vi "Ballard - 1553 Asynchronous RT Driver VI.vi"(10 "Parameters":variant, 11 "Process":refnum<class "Process.lvclass">) -> ()   [LabVIEW 2017, in "Ballard MIL-1553 Engine.lvlib"]
doc: "This VI is the Asynchronous VI for RT part."
uses:
  Ballard MIL-1553 Engine.lvlib
  <vilib>/NI/NIVS Inline Async API/_VS Inline Async API/Process/Process.lvclass
  Controls/RT Async Data.ctl
  Controls/RT Async_Map BC2RT.ctl
  <vilib>/NI Veristand/Custom Device API/Data Reference.ctl
  Controls/RT Async_Map_Type.ctl
  Controls/RT Async_Raw Values.ctl
  Controls/RT Async_Raw Values to Messages Index_Association.ctl
  Controls/RT Async_Map RT2BC.ctl
  Controls/RT Async_Map RTs Status.ctl
  Controls/RT Async_Map BC Command Channels.ctl
  <vilib>/NI Veristand/Custom Device API/Custom Device Item Ref.ctl
  Controls/RT Async_Map BC Acyclic Messages Trigger.ctl
  Controls/RT Async_Map RT Command Channels.ctl
  <vilib>/NI/NIVS Inline Async API/_VS Inline Async API/Process/Process.lvclass/Process.ctl
  <vilib>/NI/NIVS Inline Async API/_Data Access Engine/Access Type Classes/Read/Read.lvclass/Read.ctl
  <vilib>/NI/NIVS Inline Async API/_Data Access Engine/Access Type Classes/ReadWrite/ReadWrite.lvclass/ReadWrite.ctl
  <vilib>/NI/NIVS Inline Async API/_Data Access Engine/Access Type Classes/Write/Write.lvclass/Write.ctl
  <vilib>/NI/NIVS Inline Async API/_Data Access Engine/Data Access Engine/Methods/Read.Data.Detect.vi
  <vilib>/NI/NIVS Inline Async API/_Data Access Engine/Data Access Engine/Methods/ReadWrite.Data.Read.vi
  <vilib>/NI/NIVS Inline Async API/_Data Access Engine/Data Access Engine/Methods/ReadWrite.Data.Reset.vi
  <vilib>/NI/NIVS Inline Async API/_Data Access Engine/Data Access Engine/Methods/Write.Data.vi
  <vilib>/NI/NIVS Inline Async API/_Data Access Engine/Data Access Engine/Methods/Read.Data.vi
  <vilib>/NI/NIVS Inline Async API/_VS Inline Async API/Process/Data Member Access/Read Data Access.vi
  <vilib>/NI/NIVS Inline Async API/_VS Inline Async API/Error Handling Process/SubVIs/Error.ConvertArray.vi
  <vilib>/NI/NIVS Inline Async API/_Data Access Engine/Access Type Classes/Read/Read.ProcessData.Detect.vi
  <vilib>/NI/NIVS Inline Async API/_Data Access Engine/Access Type Classes/ReadWrite/ReadWrite.ProcessData.Read.vi
  <vilib>/NI/NIVS Inline Async API/_Data Access Engine/Access Type Classes/ReadWrite/ReadWrite.ProcessData.Reset.vi
  <vilib>/NI/NIVS Inline Async API/_Data Access Engine/Access Type Classes/Write/Write.ProcessData.vi
  <vilib>/NI/NIVS Inline Async API/_Data Access Engine/Access Type Classes/Read/Read.ProcessData.vi
  <vilib>/NI/NIVS Inline Async API/_Data Access Engine/Data Access Engine/Methods/Read.Lookup.vi
  <vilib>/NI/NIVS Inline Async API/_Data Access Engine/Data Access Engine/Methods/Write.Lookup.vi
  <vilib>/NI/NIVS Inline Async API/_Data Access Engine/Data Access Engine/Methods/ReadWrite.Lookup.vi
  <vilib>/NI/NIVS Inline Async API/_Data Access Engine/Data Access Engine/Data Access Engine.lvclass
  <vilib>/NI VeriStand/Custom Device API/Custom Device API.lvlib
panel:
  # "Custom Device Template\nv1.0"
  # "Use this template as a starting point for creating a custom device code module. The input controls shown here are specially named controls that the system will use to provide the device loop with data. The controls are not required for the device loop to run. For instance, if the device doesn't produce any output data, then you don't need the Device Outputs FIFO control. If you do use these controls, however, they need to have these exact names to be functional."
  # "The optional status notifier element is used to notify the RT engine of the last state of the custom device, and to indicate the device has completed execution. If this control is not used, a default No Error value is returned to the system when the device finishes execution.\n\nNote: This error state is not checked until the system shuts down. Use an output status channel to send more immediate status values to the system."
  # "This optional input can be used to send the VeriStand Engine the final status of the custom device initalization process. If this control exists on the custom device front panel, the VeriStand Engine will wait for a status update before starting up. If the custom device reports an error, that will abort the execution of the current configuration in the VeriStand Engine.\n\nThis control can be deleted if the custom device does not need to send the initialization status update."
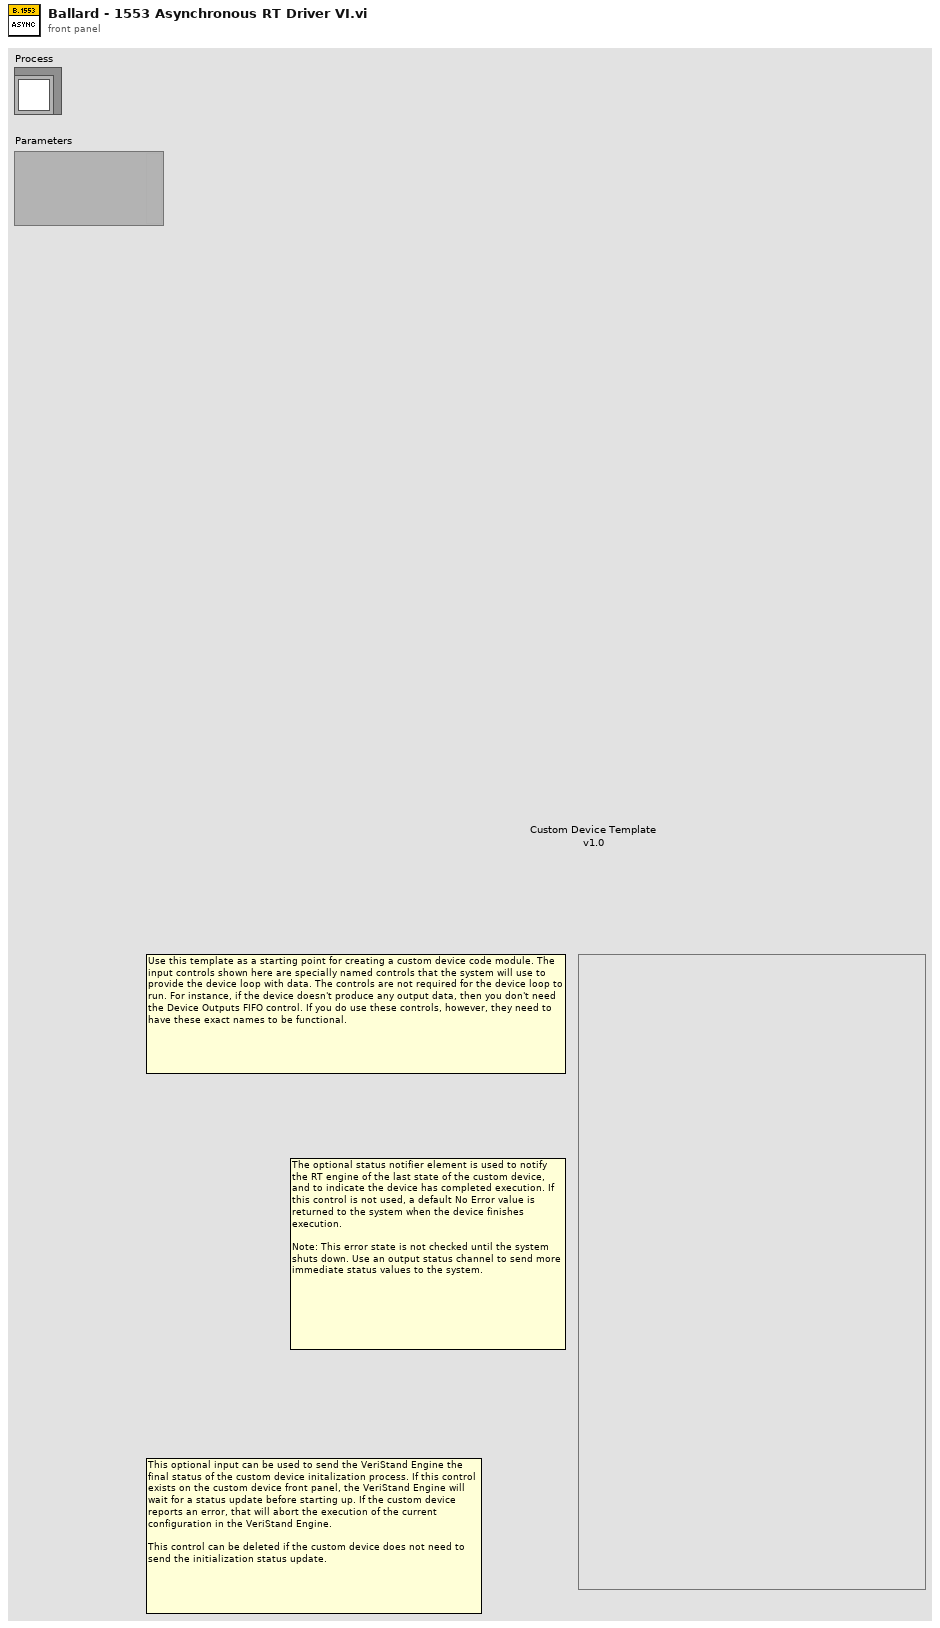
[diagram p1: front panel]
types:
  T1 = typedef "Ballard MIL-1553 Engine.lvlib/RT Async Data.ctl" = cluster{"Map (BC to RT)":T2[], "Raw Values (BC to RT)":T5, "Map (RT to ..)":T7[], "Raw Values (RT to ..)":T5, "Map (RTs Status)":T8[], "Raw Values (RTs Status)":T5, "Map (Bc Command Channels)":T9[], "MAP (BC Acyclic Messages Trigger)":T11[], "Map (RT Command Channels)":T12[], "Map (MC Rx)":T2[], "Raw Values (MC Rx)":T5, "Raw Values (MC Tx)":T5, "Map (MC Tx)":T7[]}
  T2 = typedef "Ballard MIL-1553 Engine.lvlib/RT Async_Map BC2RT.ctl" = cluster{"Channel Index":i32, "ID":i32, "Channel Data Reference":T3, "Word Index":i32, "Message Handle":u64, "Type":T4, "Word Count":i32, "First Element Index":i32}
  T3 = typedef "Custom Device API.lvlib/Data Reference.ctl" = i32
  T4 = typedef "Ballard MIL-1553 Engine.lvlib/RT Async_Map_Type.ctl" = enum16{"Word (BC to RT)", "Word (MC (Rx))", "Acyclic Message Trigger", "Word (RT to ..)", "Word (RT to RT)", "Word (MC (Tx))", "RT Status", "BC Commands", "RT Commands"}
  T5 = typedef "Ballard MIL-1553 Engine.lvlib/RT Async_Raw Values.ctl" = cluster{"Association":T6[], "Raw Values Array":u16[]}
  T6 = typedef "Ballard MIL-1553 Engine.lvlib/RT Async_Raw Values to Messages Index_Association.ctl" = cluster{"Message Index":i32, "Raw Value Index":i32}
  T7 = typedef "Ballard MIL-1553 Engine.lvlib/RT Async_Map RT2BC.ctl" = cluster{"Channel Index":i32, "ID":i32, "Word Data Reference":T3, "First element Index":i32, "rt Transfer Handle":u64, "Type":T4, "Word Count":i32}
  T8 = typedef "Ballard MIL-1553 Engine.lvlib/RT Async_Map RTs Status.ctl" = cluster{"Channel Index":i32, "ID":i32, "rt Transfer Handle":u64, "Type":T4}
  T9 = typedef "Ballard MIL-1553 Engine.lvlib/RT Async_Map BC Command Channels.ctl" = cluster{"Channel Index":i32, "ID":i32, "BC Handle":u64, "Type":T4, "BC Command Channel Ref":T10, "Command Type":enum16{"Start Command", "Stop Command"}}
  T10 = typedef "Custom Device API.lvlib/Custom Device Item Ref.ctl" = u64
  T11 = typedef "Ballard MIL-1553 Engine.lvlib/RT Async_Map BC Acyclic Messages Trigger.ctl" = cluster{"Channel Index":i32, "BC Handle":u64, "Type":T4, "Acyclic Message Trigger Channel Ref":T10, "Message Name":string}
  T12 = typedef "Ballard MIL-1553 Engine.lvlib/RT Async_Map RT Command Channels.ctl" = cluster{"Channel Index":i32, "ID":i32, "RT Handle":u64, "Type":T4, "RT Command Channel Ref":T10, "Command Type":enum16{"Start Command", "Stop Command"}}
  T13 = typedef "Data Access Engine.lvlib/Data Access Engine.lvclass/Read.DVR.ctl" = refnum<data-value>
  T14 = typedef "Data Access Engine.lvlib/Data Access Engine.lvclass/ReadWrite.DVR.ctl" = refnum<data-value>
  T15 = typedef "Data Access Engine.lvlib/Data Access Engine.lvclass/Write.DVR.ctl" = refnum<data-value>
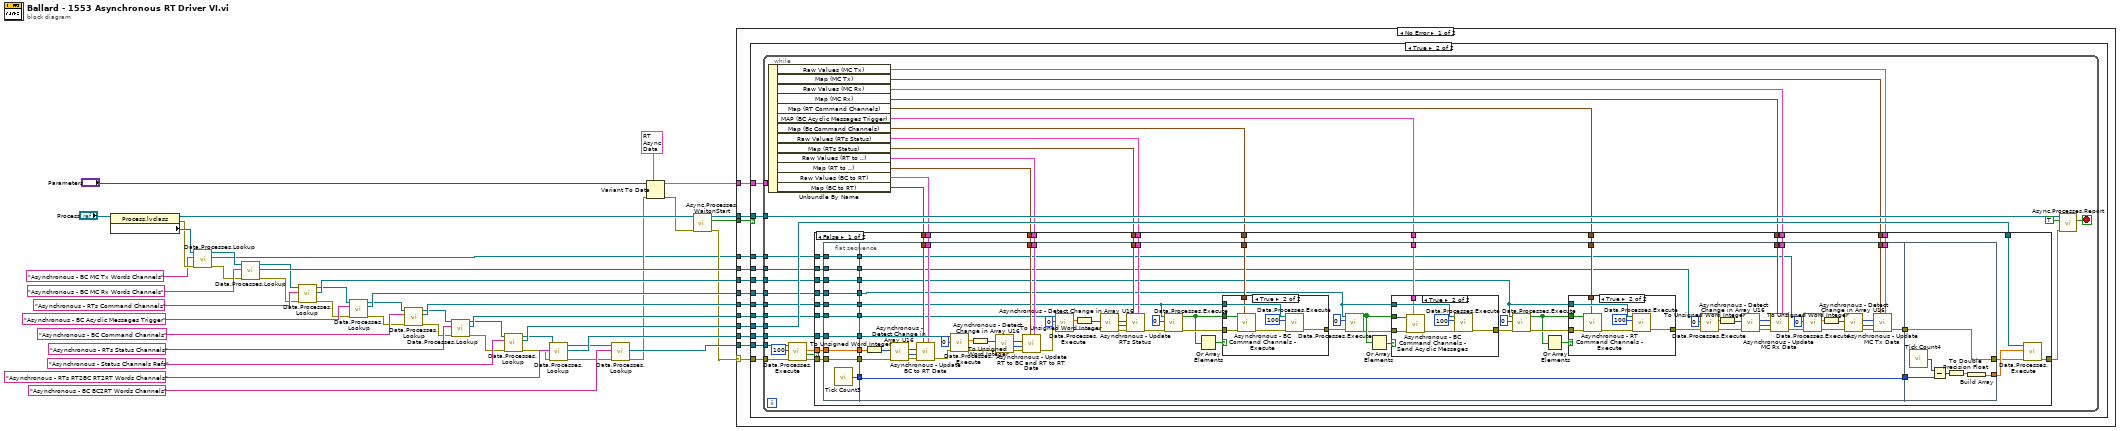
[diagram p0: block diagram]
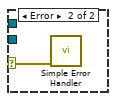
[diagram p7: hidden frame]
diagram:
  n1 = property class="Process.lvclass"(reference="Process") -> (reference out=w41:refnum<class "Process.lvclass">, error out=w5:errorcluster, "Data Member Access:Data Access"=w6:refnum<class "Data Access Engine.lvclass">)  [unwired: 1 in]
  n2 = call-poly <vilib>:"Data.Processes.Lookup.vi"("error in (no error)"=w5, "Name"="Asynchronous - BC MC Tx Words Channels", "Data Access API in"=w6) -> ("error out"=w4:errorcluster, "Ref"=w2:T13, "Data Access API out"=w3:refnum<class "Data Access Engine.lvclass">)  [unwired: 5 in, 1 out]
  n3 = call-poly <vilib>:"Data.Processes.Lookup.vi"("error in (no error)"=w4, "Name"="Asynchronous - BC MC Rx Words Channels", "Data Access API in"=w3) -> ("error out"=w7:errorcluster, "Ref"=w23:T13, "Data Access API out"=w8:refnum<class "Data Access Engine.lvclass">)  [unwired: 5 in, 1 out]
  n4 = call-poly <vilib>:"Data.Processes.Lookup.vi"("error in (no error)"=w7, "Name"="Asynchronous - RTs Command Channels", "Data Access API in"=w8) -> ("error out"=w9:errorcluster, "Ref"=w25:T14, "Data Access API out"=w10:refnum<class "Data Access Engine.lvclass">)  [unwired: 5 in, 1 out]
  n5 = call-poly <vilib>:"Data.Processes.Lookup.vi"("error in (no error)"=w9, "Name"="Asynchronous - BC Acyclic Messages Trigger", "Data Access API in"=w10) -> ("error out"=w12:errorcluster, "Ref"=w27:T14, "Data Access API out"=w11:refnum<class "Data Access Engine.lvclass">)  [unwired: 5 in, 1 out]
  n6 = call-poly <vilib>:"Data.Processes.Lookup.vi"("error in (no error)"=w12, "Name"="Asynchronous - BC Command Channels", "Data Access API in"=w11) -> ("error out"=w13:errorcluster, "Ref"=w29:T14, "Data Access API out"=w14:refnum<class "Data Access Engine.lvclass">)  [unwired: 5 in, 1 out]
  n7 = call-poly <vilib>:"Data.Processes.Lookup.vi"("error in (no error)"=w13, "Name"="Asynchronous - RTs Status Channels", "Data Access API in"=w14) -> ("error out"=w15:errorcluster, "Ref"=w31:T13, "Data Access API out"=w16:refnum<class "Data Access Engine.lvclass">)  [unwired: 5 in, 1 out]
  n8 = call-poly <vilib>:"Data.Processes.Lookup.vi"("error in (no error)"=w15, "Name"="Asynchronous - Status Channels Refs", "Data Access API in"=w16) -> ("error out"=w17:errorcluster, "Ref"=w43:T15, "Data Access API out"=w18:refnum<class "Data Access Engine.lvclass">)  [unwired: 5 in, 1 out]
  n9 = call-poly <vilib>:"Data.Processes.Lookup.vi"("error in (no error)"=w17, "Name"="Asynchronous - RTs RT2BC RT2RT Words Channels", "Data Access API in"=w18) -> ("error out"=w19:errorcluster, "Ref"=w37:T13, "Data Access API out"=w35:refnum<class "Data Access Engine.lvclass">)  [unwired: 5 in, 1 out]
  n10 = call-poly <vilib>:"Data.Processes.Lookup.vi"("error in (no error)"=w19, "Name"="Asynchronous - BC BC2RT Words Channels", "Data Access API in"=w35) -> ("error out"=w20:errorcluster, "Ref"=w44:T13)  [unwired: 5 in, 2 out]
  n11 = Variant To Data(error in=w20, type=T1 {"Map (BC to RT)"=[], "Raw Values (BC to RT)"={"Association"=[], "Raw Values Array"=[]}, "Map (RT to ..)"=[], "Raw Values (RT to ..)"={"Association"=[], "Raw Values Array"=[]}, "Map (RTs Status)"=[], "Raw Values (RTs Status)"={"Association"=[], "Raw Values Array"=[]}, "Map (Bc Command Channels)"=[], "MAP (BC Acyclic Messages Trigger)"=[], "Map (RT Command Channels)"=[], "Map (MC Rx)"=[], "Raw Values (MC Rx)"={"Association"=[], "Raw Values Array"=[]}, "Raw Values (MC Tx)"={"Association"=[], "Raw Values Array"=[]}, "Map (MC Tx)"=[]} ("RT Async Data"), Variant="Parameters") -> (data=w36:T1, error out=w21:errorcluster)
  n12 = call <vilib>:"Async.Processes.WaitonStart.vi"("error in (no error)"=w21, "Process"=w41) -> ("error out"=w22:errorcluster, "Execute"=w46:bool, "Process out"=w45:refnum<class "Process.lvclass">)  [unwired: 7 in]
  n13 = case shown="No Error" w22 {
    selector: w22 -> [w55 w258]
    tunnel: w46 -> [w59 _]
    tunnel: w45 -> [w58 _]
    tunnel: w43 -> [w57 _]
    tunnel: w44 -> [w56 _]
    tunnel: w36 -> [w54 _]
    tunnel: w37 -> [w53 _]
    tunnel: w31 -> [w52 _]
    tunnel: w29 -> [w51 _]
    tunnel: w27 -> [w50 _]
    tunnel: w25 -> [w49 _]
    tunnel: w23 -> [w48 _]
    tunnel: w2 -> [w47 _]
    frame No Error {
      n14 = case shown="True" w59 {
        tunnel: w55 -> [_ w68]
        tunnel: w58 -> [_ w69]
        tunnel: w56 -> [_ w71]
        tunnel: w57 -> [_ w70]
        tunnel: w54 -> [_ w67]
        tunnel: w53 -> [_ w66]
        tunnel: w52 -> [_ w65]
        tunnel: w51 -> [_ w64]
        tunnel: w50 -> [_ w63]
        tunnel: w49 -> [_ w62]
        tunnel: w48 -> [_ w61]
        tunnel: w47 -> [_ w60]
        frame False {
        }
        frame True {
          n15 = while {
            tunnel: w68 -> [w99]
            tunnel: w69 -> [w103]
            tunnel: w71 -> [w101]
            tunnel: w70 -> [w100]
            tunnel: w67 -> [w96]
            tunnel: w66 -> [w95]
            tunnel: w65 -> [w88]
            tunnel: w64 -> [w85]
            tunnel: w63 -> [w83]
            tunnel: w62 -> [w81]
            tunnel: w61 -> [w79]
            tunnel: w60 -> [w74]
            stop <- w102 stop-if-true
            n16 = Unbundle By Name(w96) -> ("Raw Values (MC Tx)"=w72:T5, "Map (MC Tx)"=w73:T7[], "Raw Values (MC Rx)"=w76:T5, "Map (MC Rx)"=w75:T2[], "Map (RT Command Channels)"=w80:T12[], "MAP (BC Acyclic Messages Trigger)"=w82:T11[], "Map (Bc Command Channels)"=w84:T9[], "Raw Values (RTs Status)"=w86:T5, "Map (RTs Status)"=w87:T8[], "Raw Values (RT to ..)"=w91:T5, "Map (RT to ..)"=w92:T7[], "Raw Values (BC to RT)"=w89:T5, "Map (BC to RT)"=w90:T2[])
            n17 = call-poly <vilib>:"Data.Processes.Execute.vi"("error in (no error)"=w99, "timeout ms"=100, "Ref"=w101) -> ("error out"=w97:errorcluster, "Timeout?"=w94:bool, "Values"=w98:dbl[])  [unwired: 6 in]
            n18 = case shown="False" w94 {
              tunnel: w100 -> [w136 _]
              tunnel: [w135 w257] -> w78
              tunnel: w98 -> [w134 _]
              tunnel: w97 -> [w133 w257]
              tunnel: w95 -> [w131 _]
              tunnel: w92 -> [w130 _]
              tunnel: w91 -> [w129 _]
              tunnel: w90 -> [w128 _]
              tunnel: w89 -> [w127 _]
              tunnel: w88 -> [w126 _]
              tunnel: w87 -> [w124 _]
              tunnel: w86 -> [w123 _]
              tunnel: w85 -> [w122 _]
              tunnel: w84 -> [w119 _]
              tunnel: w83 -> [w118 _]
              tunnel: w82 -> [w116 _]
              tunnel: w81 -> [w115 _]
              tunnel: w80 -> [w113 _]
              tunnel: w79 -> [w112 _]
              tunnel: w76 -> [w109 _]
              tunnel: w75 -> [w108 _]
              tunnel: w74 -> [w107 _]
              tunnel: w73 -> [w105 _]
              tunnel: w72 -> [w104 _]
              frame False {
                n19 = flat-sequence {
                  tunnel: w134 -> [w150]
                  tunnel: w133 -> [w151]
                  tunnel: [w151] -> w141
                  tunnel: [w150] -> w140
                  tunnel: [w149] -> w139
                  tunnel: w131 -> [w148]
                  tunnel: [w148] -> w138
                  tunnel: w126 -> [w147]
                  tunnel: [w147] -> w125
                  tunnel: w122 -> [w146]
                  tunnel: [w146] -> w121
                  tunnel: w118 -> [w145]
                  tunnel: [w145] -> w117
                  tunnel: w115 -> [w144]
                  tunnel: [w144] -> w114
                  tunnel: w112 -> [w143]
                  tunnel: [w143] -> w111
                  tunnel: w107 -> [w142]
                  tunnel: [w142] -> w106
                  tunnel: w141 -> [w221]
                  tunnel: w140 -> [w220]
                  tunnel: w139 -> [w226]
                  tunnel: [w226] -> w137
                  tunnel: w138 -> [w225]
                  tunnel: w130 -> [w224]
                  tunnel: w129 -> [w223]
                  tunnel: w128 -> [w216]
                  tunnel: w127 -> [w215]
                  tunnel: w125 -> [w213]
                  tunnel: w124 -> [w212]
                  tunnel: w123 -> [w211]
                  tunnel: w121 -> [w210]
                  tunnel: w119 -> [w209]
                  tunnel: w117 -> [w208]
                  tunnel: w116 -> [w207]
                  tunnel: w114 -> [w206]
                  tunnel: w113 -> [w205]
                  tunnel: w111 -> [w204]
                  tunnel: [w155] -> w110
                  tunnel: w109 -> [w165]
                  tunnel: w108 -> [w164]
                  tunnel: w106 -> [w154]
                  tunnel: w105 -> [w153]
                  tunnel: w104 -> [w152]
                  tunnel: w137 -> [w256]
                  tunnel: [w252] -> w132
                  tunnel: [w251] -> w120
                  tunnel: w110 -> [w251]
                  frame #0 {
                    n20 = call "Tick Count3"() -> ("Tick Count(uSec)"=w149:u32)
                  }
                  frame #1 {
                    n21 = To Unsigned Word Integer(number=w220) -> (unsigned 16bit integer=w222:u16[])
                    n22 = call "Asynchronous - Detect Change in Array U16.vi"("Error (in)"=w221, "Data (in)"=w222) -> ("Error (out)"=w219:errorcluster, "Indexes"=w217:i32[], "Data (out)"=w218:u16[])  [unwired: 7 in]
                    n23 = call "Asynchronous - Update BC to RT Data.vi"("Raw Values (BC to RT)"=w215, "Map (BC to RT)"=w216, "Error (in)"=w219, "Updated FIFO Index []"=w217, "U16 []"=w218) -> ("Error (out)"=w214:errorcluster)  [unwired: 6 in]
                    n24 = call-poly <vilib>:"Data.Processes.Execute.vi"("error in (no error)"=w214, "timeout ms"=0, "Ref"=w225) -> ("error out"=w200:errorcluster, "Values"=w202:dbl[])  [unwired: 5 in, 2 out]
                    n25 = To Unsigned Word Integer(number=w202) -> (unsigned 16bit integer=w201:u16[])
                    n26 = call "Asynchronous - Detect Change in Array U16.vi"("Error (in)"=w200, "Data (in)"=w201) -> ("Error (out)"=w199:errorcluster, "Indexes"=w198:i32[], "Data (out)"=w197:u16[])  [unwired: 7 in]
                    n27 = call "Asynchronous - Update RT to BC and RT to RT Data.vi"("Raw Values (RT to BC)"=w223, "Map (RT to BC)"=w224, "Error (in)"=w199, "Updated FIFO Index []"=w198, "U16 []"=w197) -> ("Error (out)"=w196:errorcluster)  [unwired: 6 in]
                    n28 = call-poly <vilib>:"Data.Processes.Execute.vi"("error in (no error)"=w196, "timeout ms"=0, "Ref"=w213) -> ("error out"=w192:errorcluster, "Values"=w194:dbl[])  [unwired: 5 in, 2 out]
                    n29 = To Unsigned Word Integer(number=w194) -> (unsigned 16bit integer=w193:u16[])
                    n30 = call "Asynchronous - Detect Change in Array U16.vi"("Error (in)"=w192, "Data (in)"=w193) -> ("Error (out)"=w191:errorcluster, "Indexes"=w189:i32[], "Data (out)"=w190:u16[])  [unwired: 7 in]
                    n31 = call "Asynchronous - Update RTs Status.vi"("Raw Values (RTs Status)"=w211, "Map (RTs Status)"=w212, "Error (in)"=w191, "Updated FIFO Index []"=w189, "U16 []"=w190) -> ("Error (out)"=w187:errorcluster)  [unwired: 6 in]
                    n32 = call-poly <vilib>:"Data.Processes.Execute.vi"("error in (no error)"=w187, "timeout ms"=0, "Ref"=w210) -> ("error out"=w185:errorcluster, "Detect?"=w184:bool[])  [unwired: 5 in, 2 out]
                    n33 = Or Array Elements(Boolean array=w184) -> (logical OR=w186:bool)
                    n34 = case shown="True" w186 {
                      tunnel: w185 -> [w243 w247]
                      tunnel: w210 -> [_ w249]
                      tunnel: w184 -> [_ w245]
                      tunnel: [w243 w248] -> w183
                      tunnel: w209 -> [_ w244]
                      frame False {
                      }
                      frame True {
                        n35 = call "Asynchronous - BC Command Channels - Execute.vi"("Map (Bc Command Channels)"=w244, "Error (in)"=w247, "Changes?"=w245) -> ("Error (out)"=w246:errorcluster)  [unwired: 8 in]
                        n36 = call-poly <vilib>:"Data.Processes.Execute.vi"("error in (no error)"=w246, "timeout ms"=100, "Ref"=w249) -> ("error out"=w248:errorcluster)  [unwired: 7 in, 1 out]
                      }
                    }
                    n37 = call-poly <vilib>:"Data.Processes.Execute.vi"("error in (no error)"=w183, "timeout ms"=0, "Ref"=w208) -> ("error out"=w180:errorcluster, "Detect?"=w181:bool[])  [unwired: 5 in, 2 out]
                    n38 = Or Array Elements(Boolean array=w181) -> (logical OR=w179:bool)
                    n39 = case shown="True" w179 {
                      tunnel: w180 -> [w235 w239]
                      tunnel: w208 -> [_ w241]
                      tunnel: w181 -> [_ w237]
                      tunnel: [w235 w240] -> w175
                      tunnel: w207 -> [_ w236]
                      frame False {
                      }
                      frame True {
                        n40 = call "Asynchronous - BC Command Channels - Send Acyclic Messages.vi"("Map (Bc Acyclic Messages Trigger)"=w236, "Error (in)"=w239, "Changes?"=w237) -> ("Error (out)"=w238:errorcluster)  [unwired: 8 in]
                        n41 = call-poly <vilib>:"Data.Processes.Execute.vi"("error in (no error)"=w238, "timeout ms"=100, "Ref"=w241) -> ("error out"=w240:errorcluster)  [unwired: 7 in, 1 out]
                      }
                    }
                    n42 = call-poly <vilib>:"Data.Processes.Execute.vi"("error in (no error)"=w175, "timeout ms"=0, "Ref"=w206) -> ("error out"=w177:errorcluster, "Detect?"=w176:bool[])  [unwired: 5 in, 2 out]
                    n43 = Or Array Elements(Boolean array=w176) -> (logical OR=w174:bool)
                    n44 = case shown="True" w174 {
                      tunnel: w177 -> [w227 w231]
                      tunnel: w206 -> [_ w233]
                      tunnel: w176 -> [_ w229]
                      tunnel: [w227 w232] -> w173
                      tunnel: w205 -> [_ w228]
                      frame False {
                      }
                      frame True {
                        n45 = call "Asynchronous - RT Command Channels - Execute.vi"("Map (RT Command Channels)"=w228, "Error (in)"=w231, "Changes?"=w229) -> ("Error (out)"=w230:errorcluster)  [unwired: 8 in]
                        n46 = call-poly <vilib>:"Data.Processes.Execute.vi"("error in (no error)"=w230, "timeout ms"=100, "Ref"=w233) -> ("error out"=w232:errorcluster)  [unwired: 7 in, 1 out]
                      }
                    }
                    n47 = call-poly <vilib>:"Data.Processes.Execute.vi"("error in (no error)"=w173, "timeout ms"=0, "Ref"=w204) -> ("error out"=w170:errorcluster, "Values"=w171:dbl[])  [unwired: 5 in, 2 out]
                    n48 = To Unsigned Word Integer(number=w171) -> (unsigned 16bit integer=w169:u16[])
                    n49 = call "Asynchronous - Detect Change in Array U16.vi"("Error (in)"=w170, "Data (in)"=w169) -> ("Error (out)"=w168:errorcluster, "Indexes"=w167:i32[], "Data (out)"=w166:u16[])  [unwired: 7 in]
                    n50 = call "Asynchronous - Update MC Rx Data.vi"("Raw Values (MC Rx)"=w165, "Map (MC Rx)"=w164, "Error (in)"=w168, "Updated FIFO Index []"=w167, "U16 []"=w166) -> ("Error (out)"=w156:errorcluster)  [unwired: 6 in]
                    n51 = call-poly <vilib>:"Data.Processes.Execute.vi"("error in (no error)"=w156, "timeout ms"=0, "Ref"=w154) -> ("error out"=w159:errorcluster, "Values"=w158:dbl[])  [unwired: 5 in, 2 out]
                    n52 = To Unsigned Word Integer(number=w158) -> (unsigned 16bit integer=w160:u16[])
                    n53 = call "Asynchronous - Detect Change in Array U16.vi"("Error (in)"=w159, "Data (in)"=w160) -> ("Error (out)"=w161:errorcluster, "Indexes"=w162:i32[], "Data (out)"=w163:u16[])  [unwired: 7 in]
                    n54 = call "Asynchronous - Update MC Tx Data.vi"("Raw Values (MC Tx)"=w152, "Map (MC Tx)"=w153, "Error (in)"=w161, "Updated FIFO Index []"=w162, "U16 []"=w163) -> ("Error (out)"=w155:errorcluster)  [unwired: 6 in]
                  }
                  frame #2 {
                    n55 = call "Tick Count4"() -> ("Tick Count(uSec)"=w255:u32)
                    n56 = Subtract(x=w255, y=w256) -> (x-y=w254:u32)
                    n57 = To Double Precision Float(number=w254) -> (double precision float=w253:dbl)
                    n58 = Build Array(w253) -> (w252:dbl[])
                  }
                }
                n59 = call-poly <vilib>:"Data.Processes.Execute.vi"("error in (no error)"=w120, "Values"=w132, "Ref"=w136) -> ("error out"=w135:errorcluster)  [unwired: 8 in]
              }
              frame True {
              }
            }
            n60 = call <vilib>:"Async.Processes.Report.vi"("Error"=w78, "Stop Async on Error?"=TRUE, "Process in"=w103) -> ("Stop"=w102:bool)  [unwired: 7 in, 1 out]
          }
        }
      }
    }
    frame Error {
      n61 = call <vilib>:"Simple Error Handler.vi"("error in (no error)"=w258) -> ()  [unwired: 4 in, 5 out]
    }
  }
